vi "求和取余校验.vi"(11 "字符串":string) -> (3 "求和校验码":string)   [LabVIEW 2014]
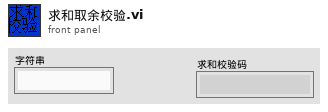
[diagram p1: front panel]
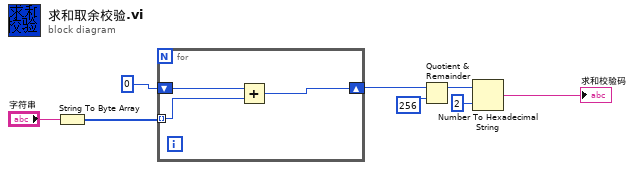
[diagram p0: block diagram]
diagram:
  n1 = String To Byte Array(string="字符串") -> (unsigned byte array=w8:u8[])
  n2 = for {
    tunnel: w8 -> [w10] mode=indexing
    shift-right: [w9] -> w6
    shift-left: u32 0 -> [w11]
    n3 = Add(x=w11, y=w10) -> (x+y=w9:u32)
  }
  n4 = Quotient & Remainder(x=w6, y=u32 256) -> (x-y*floor(x/y)=w4:u32)  [unwired: 1 out]
  n5 = Number To Hexadecimal String(1:i16 2 ("宽度(-)"), 2:w4) -> (0:→"求和校验码":string)
